vi "read_Pressure_limit_file.vi"() -> (1 "LO":dbl[](array[numeric]), 2 "HI":dbl[](array[numeric]), 3 "Pressure_names":string[](array[string]))   [LabVIEW 2013]
uses:
  <vilib>/Utility/file.llb/Read From Spreadsheet File (string).vi
panel:
  out "all rows":string[][](array[string])
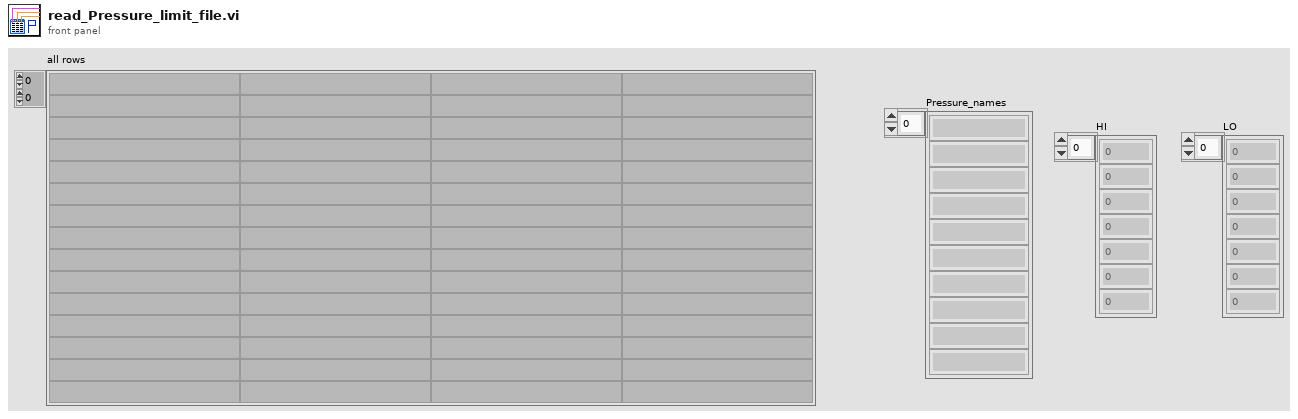
[diagram p1: front panel]
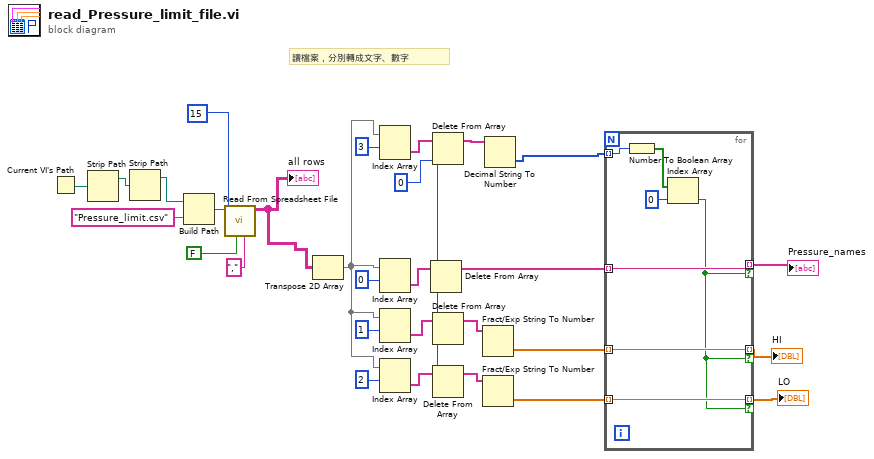
[diagram p0: block diagram]
diagram:
  w16 = 0 ("index")
  # "讀檔案，分別轉成文字、數字"
  n1 = Current VI's Path() -> (path=w24:path)
  n2 = Strip Path(path=w24) -> (stripped path=w25:path)  [unwired: 1 out]
  n3 = Strip Path(path=w25) -> (stripped path=w27:path)  [unwired: 1 out]
  n4 = Build Path(base path=w27, name or relative path="Pressure_limit.csv") -> (appended path=w28:path)
  n5 = call-poly <vilib>:"Read From Spreadsheet File.vi"("delimiter (\\t)"="," ("delimiter (\\t)"), "transpose (no:F)"=FALSE, "start of read offset (chars.:0)"=15, "file path (dialog if empty)"=w28) -> ("all rows"=w4:string[][])  [unwired: 3 in, 4 out]
  "all rows" <- w4
  n6 = Transpose 2D Array(2D array=w4) -> (transposed array=w15:string[][])
  n7 = Index Array(array=w15, index (row)=3) -> (element=w13:string[])  [unwired: 1 in]
  n8 = Index Array(array=w15, index (row)=0) -> (element=w8:string[])  [unwired: 1 in]
  n9 = Index Array(array=w15, index (row)=1) -> (element=w9:string[])  [unwired: 1 in]
  n10 = Index Array(array=w15, index (row)=2) -> (element=w10:string[])  [unwired: 1 in]
  n11 = Delete From Array(array=w8, index=w16) -> (array with subset deleted=w21:string[])  [unwired: 1 in, 1 out]
  n12 = Delete From Array(array=w13, index=w16) -> (array with subset deleted=w17:string[])  [unwired: 1 in, 1 out]
  n13 = Delete From Array(array=w9, index=w16) -> (array with subset deleted=w11:string[])  [unwired: 1 in, 1 out]
  n14 = Delete From Array(array=w10, index=w16) -> (array with subset deleted=w12:string[])  [unwired: 1 in, 1 out]
  n15 = Fract/Exp String To Number(string=w11) -> (number=w19:dbl[])  [unwired: 3 in, 1 out]
  n16 = Fract/Exp String To Number(string=w12) -> (number=w20:dbl[])  [unwired: 3 in, 1 out]
  n17 = Decimal String To Number(string=w17) -> (number=w18:i32[])  [unwired: 2 in, 1 out]
  n18 = for {
    tunnel: w18 -> [w36] mode=indexing
    tunnel: w19 -> [w35] mode=indexing
    tunnel: [w35] -> w2 mode=indexing if=w30
    tunnel: [w34] -> w1 mode=indexing if=w30
    tunnel: w20 -> [w34] mode=indexing
    tunnel: [w31] -> w3 mode=indexing if=w30
    tunnel: w21 -> [w31] mode=indexing
    n19 = Number To Boolean Array(number=w36) -> (Boolean array=w32:bool[])
    n20 = Index Array(array=w32, index=0) -> (element=w30:bool)
  }
  "Pressure_names" <- w3
  "HI" <- w2
  "LO" <- w1
